vi "Get Node (TreePath).vi"(8 "error in (no error)":errorcluster, 10 "Path":refnum<class "TreePath.lvclass">, 11 "Tree in":refnum<class "Tree.lvclass">) -> (0 "error out":errorcluster, 2 "Node out":refnum<class "TreeNode.lvclass">, 3 "Tree out":refnum<class "Tree.lvclass">)   [LabVIEW 2013, in "MDSplus.lvlib" / "Tree.lvclass"]
doc: "Return the TreeNode for the data itemspecified by the passed TreePath instance."
uses:
  <vilib>/MDSplus/Classes/Tree_Class/Tree.lvclass
  <vilib>/MDSplus/Classes/Data_Class/TreeNode_Class/TreePath_Class/TreePath.lvclass
  <vilib>/MDSplus/Classes/Data_Class/TreeNode_Class/TreeNode.lvclass
  <vilib>/MDSplus/Classes/Data_Class/Data.lvclass
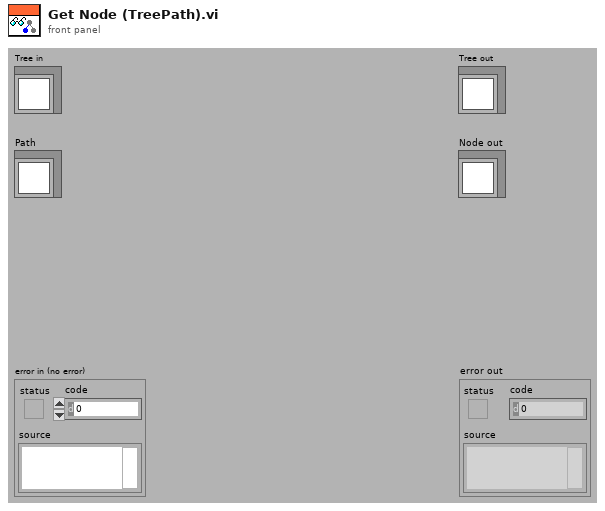
[diagram p1: front panel]
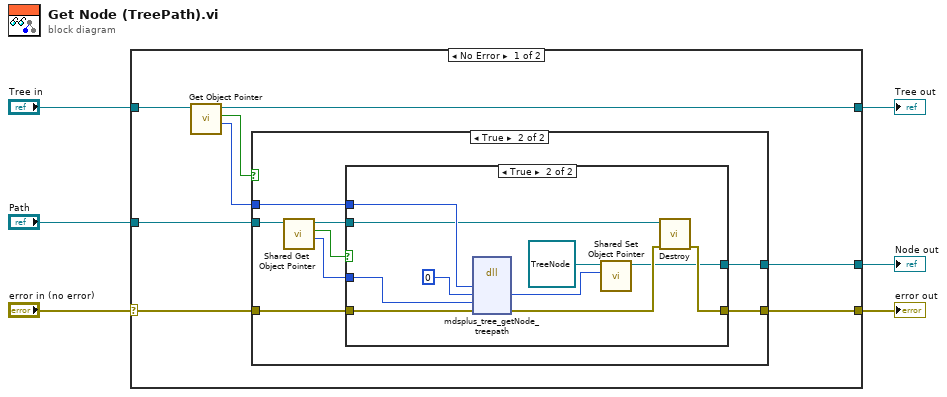
[diagram p0: block diagram]
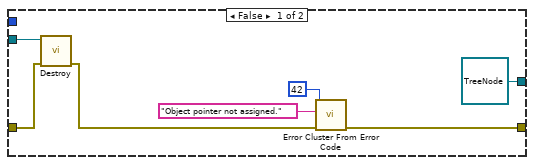
[diagram p2: hidden frame]
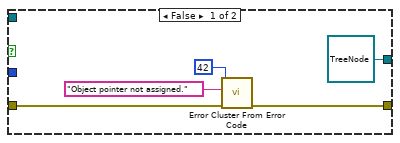
[diagram p3: hidden frame]
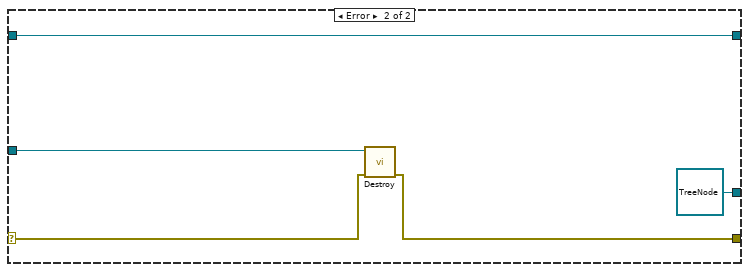
[diagram p4: hidden frame]
diagram:
  n1 = case shown="No Error" "error in (no error)" {
    selector: "error in (no error)" -> [w10 w47]
    tunnel: [w9 w46] -> w5
    tunnel: [w8 w49] -> w3
    tunnel: "Tree in" -> [w14 w49]
    tunnel: "Path" -> [w13 w48]
    tunnel: [w7 refnum<class "TreeNode.lvclass"> refnum ("Data out")] -> w1
    frame No Error {
      n2 = call-dynamic "Get Object Pointer.vi"("Tree in"=w14) -> ("Object Pointer"=w11:i64, "Assigned object pointer?"=w12:bool, "Tree out"=w8:refnum<class "Tree.lvclass">)  [unwired: 8 in]
      n3 = case shown="True" w12 {
        tunnel: w13 -> [w18 w29]
        tunnel: w11 -> [_ w26]
        tunnel: w10 -> [w17 w25]
        tunnel: [w19 w24] -> w9
        tunnel: [refnum<class "TreeNode.lvclass"> refnum ("Data out") w22] -> w7
        frame False {
          n4 = call-dynamic "Destroy.vi"("error in (no error)"=w17, "TreePath in"=w18) -> ("error out"=w16:errorcluster)  [unwired: 9 in]
          n5 = call <vilib>:"Error Cluster From Error Code.vi"("error in (no error)"=w16, "error message (\"\")"="Object pointer not assigned." ("error message (\"\")"), "error code (0)"=42) -> ("error out"=w19:errorcluster)  [unwired: 6 in]
        }
        frame True {
          n6 = call <vilib>:"Shared Get Object Pointer.vi"("Data in"=w29) -> ("Object Pointer"=w27:i64, "Assigned object pointer?"=w28:bool, "Data out"=w23:refnum<class "TreePath.lvclass">)  [unwired: 8 in]
          n7 = case shown="True" w28 {
            tunnel: w27 -> [_ w43]
            tunnel: w26 -> [_ w44]
            tunnel: w25 -> [w32 w42]
            tunnel: [w31 w39] -> w24
            tunnel: w23 -> [_ w41]
            tunnel: [refnum<class "TreeNode.lvclass"> refnum ("Data out") w35] -> w22
            frame False {
              n8 = call <vilib>:"Error Cluster From Error Code.vi"("error in (no error)"=w32, "error message (\"\")"="Object pointer not assigned." ("error message (\"\")"), "error code (0)"=42) -> ("error out"=w31:errorcluster)  [unwired: 6 in]
            }
            frame True {
              n9 = dll-call lib="MDSobjectsLVShr" fn="mdsplus_tree_getNode_treepath"("lvTreePtr"=w44, "lvTreeNodePtrOut"=i64 0, "lvTreePathPtrIn"=w43, "error"=w42) -> ("lvTreeNodePtrOut"=w36:i64, "error"=w40:errorcluster)  [unwired: 6 in, 2 out]
              n10 = call <vilib>:"Shared Set Object Pointer.vi"("Object Pointer"=w36, "Data in"=refnum<class "TreeNode.lvclass"> refnum ("TreeNode")) -> ("Data out"=w35:refnum<class "TreeNode.lvclass">)  [unwired: 9 in]
              n11 = call-dynamic "Destroy.vi"("error in (no error)"=w40, "TreePath in"=w41) -> ("error out"=w39:errorcluster)  [unwired: 9 in]
            }
          }
        }
      }
    }
    frame Error {
      n12 = call-dynamic "Destroy.vi"("error in (no error)"=w47, "TreePath in"=w48) -> ("error out"=w46:errorcluster)  [unwired: 9 in]
    }
  }
  "error out" <- w5
  "Tree out" <- w3
  "Node out" <- w1
